vi "EnqueueElement.vi"(7 "Command":T2, 8 "error in (no error)":errorcluster, 9 "Settings":T4, 10 "ImageInfo":T1, 11 "XRefnum":refnum<vi>) -> (0 "error out":errorcluster)   [LabVIEW 2019, in "AnimatorXControl.xctl"]
uses:
  AnimatorXControl.xctl
  AnimatorSettings.ctl
  QueueElement.ctl
  AnimatorCommand.ctl
panel:
  in  "QueueElement":T3
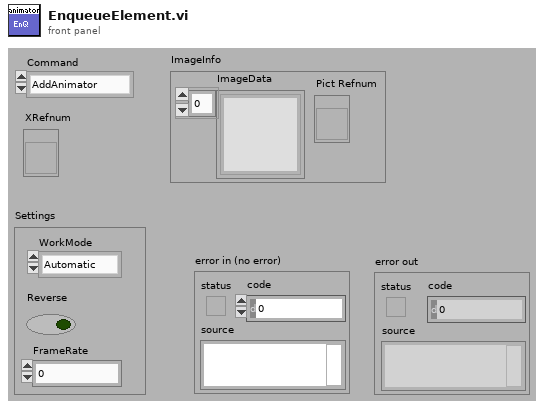
[diagram p1: front panel]
types:
  T1 = cluster{"ImageData":picture[], "Pict Refnum":refnum<vi>}
  T2 = typedef "AnimatorXControl.xctl/AnimatorCommand.ctl" = enum16{"AddAnimator", "RemoveAnimator", "Settings"}
  T3 = typedef "AnimatorXControl.xctl/QueueElement.ctl" = cluster{"Settings":T4, "Command":T2, "ImageInfo":cluster{"ImageData":picture[], "Pict Refnum":refnum<vi>}, "XRefnum":refnum<vi>}
  T4 = typedef "AnimatorXControl.xctl/AnimatorSettings.ctl" = cluster{"Reverse":bool, "FrameRate":dbl, "WorkMode":enum16{"Automatic", "UseValue"}}
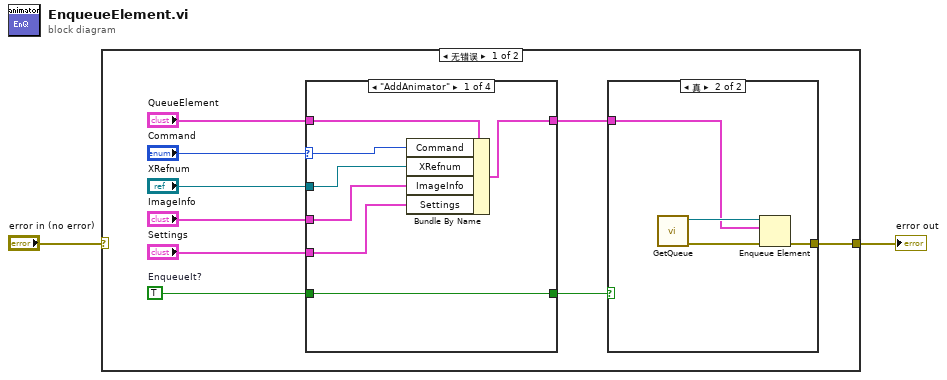
[diagram p0: block diagram]
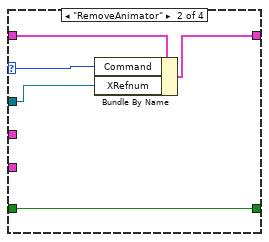
[diagram p3: hidden frame]
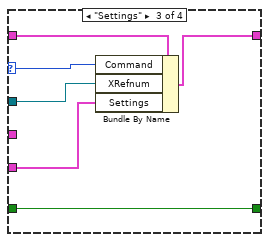
[diagram p4: hidden frame]
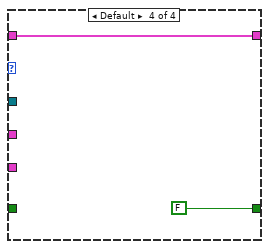
[diagram p5: hidden frame]
diagram:
  n1 = case shown="无错误" "error in (no error)" {
    selector: "error in (no error)" -> [_ w36]
    tunnel: [w8 w36] -> w2
    frame No Error {
      w11 = TRUE  # EnqueueIt?
      n2 = case shown="\"AddAnimator\"" "Command" {
        selector: "Command" -> [w18 w24 w29 _]
        tunnel: "QueueElement" -> [w22 w27 w33 w35]
        tunnel: [w21 w26 w31 w35] -> w9
        tunnel: "Settings" -> [w19 _ w32 _]
        tunnel: w11 -> [w20 w25 w30 _]
        tunnel: [w20 w25 w30 FALSE] -> w10
        tunnel: "XRefnum" -> [w17 w23 w28 _]
        tunnel: "ImageInfo" -> [w16 _ _ _]
        frame "AddAnimator" {
          n3 = Bundle By Name(cluster=w22, "Command"=w18, "XRefnum"=w17, "ImageInfo"=w16, "Settings"=w19) -> (w21:T3)
        }
        frame "RemoveAnimator" {
          n4 = Bundle By Name(cluster=w27, "Command"=w24, "XRefnum"=w23) -> (w26:T3)
        }
        frame "Settings" {
          n5 = Bundle By Name(cluster=w33, "Command"=w29, "XRefnum"=w28, "Settings"=w32) -> (w31:T3)
        }
        frame Default {
        }
      }
      n6 = case shown="真" w10 {
        tunnel: w9 -> [_ w14]
        tunnel: [_ w12] -> w8
        frame False {
        }
        frame True {
          n7 = call "GetQueue.vi"() -> ("error out"=w13:errorcluster, "queue out"=w15:refnum<queue>)  [unwired: 10 in]
          n8 = Enqueue Element(queue=w15, element=w14, error in (no error)=w13) -> (error out=w12:errorcluster)  [unwired: 1 in, 2 out]
        }
      }
    }
    frame Error {
    }
  }
  "error out" <- w2
